vi "Create Wheel Angular Velocity Row.vi"(8 "error in (no error)":errorcluster, 10 "steering angle (rad)":dbl, 11 "mecanum wheel in":refnum<class "NI_Robotics_Mecanum Wheel.lvclass">) -> (0 "error out":errorcluster, 2 "wheel angular velocity row":dbl[](array[numeric]), 3 "mecanum wheel out":refnum<class "NI_Robotics_Mecanum Wheel.lvclass">)   [LabVIEW 2017, in "NI_Robotics_Mecanum Wheel.lvclass"]
uses:
  <vilib>/robotics/Steering/Mecanum Wheel/NI_Robotics_Mecanum Wheel.lvclass
  c:/Program Files (x86)/National Instruments/LabVIEW 2017/vi.lib/robotics/Steering/Wheel/NI_Robotics_Wheel.lvclass
  <vilib>/robotics/Steering/Wheel/NI_Robotics_Wheel.lvclass/NI_Robotics_Wheel.ctl
  <vilib>/robotics/Steering/Mecanum Wheel/NI_Robotics_Mecanum Wheel.lvclass/NI_Robotics_Mecanum Wheel.ctl
  <vilib>/robotics/Steering/Wheel/NI_Robotics_Wheel.lvclass
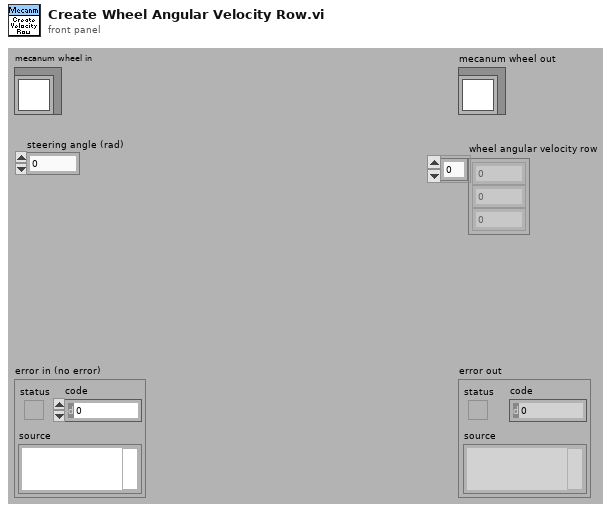
[diagram p1: front panel]
types:
  T1 = typedef "NI_Matrix.lvlib/RealMatrix.ctl" = dbl[][]
  T2 = typedef "NI_Robotics_Mecanum Wheel.lvclass/Roller Orientation.ctl" = u16
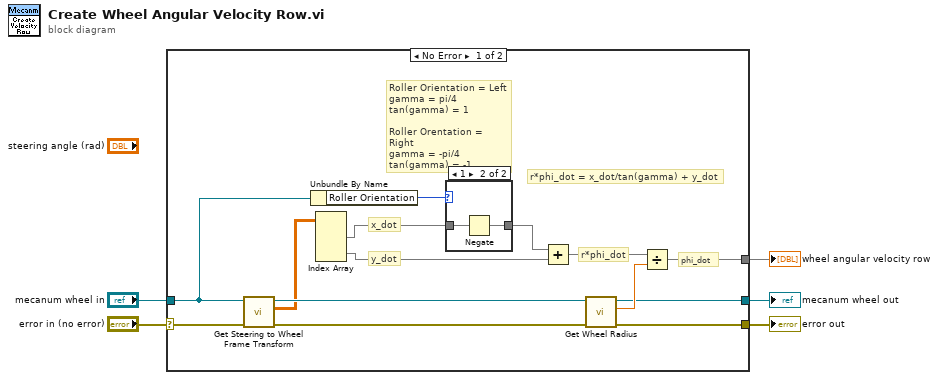
[diagram p0: block diagram]
diagram:
  n1 = case shown="No Error" "error in (no error)" {
    selector: "error in (no error)" -> [w8 w24]
    tunnel: [w15 w24] -> w4
    tunnel: "mecanum wheel in" -> [w10 w23]
    tunnel: [w14 w23] -> w2
    tunnel: [w16 _] -> w1
    frame No Error {
      # "r*phi_dot = x_dot/tan(gamma) + y_dot"
      # "phi_dot"
      # "r*phi_dot"
      # "Roller Orientation = Left\ngamma = pi/4\ntan(gamma) = 1\n\nRoller Orentation = Right\ngamma = -pi/4\ntan(gamma) = -1"
      # "y_dot"
      # "x_dot"
      n2 = call <vilib>:"Get Steering to Wheel Frame Transform.vi"("error in (no error)"=w8, "wheel in"=w10) -> ("error out"=w7:errorcluster, "steering to wheel frame transform"=w6:T1, "wheel out"=w9:refnum<class "NI_Robotics_Mecanum Wheel.lvclass">)  [unwired: 7 in]
      n3 = Unbundle By Name(w10) -> ("Roller Orientation"=w12:T2)
      n4 = Index Array(array=w6) -> (element #1=w13:dbl[], element #2=w19:dbl[])  [unwired: 4 in]
      n5 = case shown="1" w12 {
        tunnel: w13 -> [w20 w22]
        tunnel: [w20 w21] -> w11
        frame 0, Default {
        }
        frame 1 {
          n6 = Negate(x=w22) -> (-x=w21:dbl[])
        }
      }
      n7 = Add(x=w11, y=w19) -> (x+y=w18:dbl[])
      n8 = call <vilib>:"Get Wheel Radius.vi"("error in (no error)"=w7, "wheel in"=w9) -> ("error out"=w15:errorcluster, "wheel radius"=w17:dbl, "wheel out"=w14:refnum<class "NI_Robotics_Mecanum Wheel.lvclass">)  [unwired: 7 in]
      n9 = Divide(x=w18, y=w17) -> (x/y=w16:dbl[])
    }
    frame Error {
    }
  }
  "error out" <- w4
  "mecanum wheel out" <- w2
  "wheel angular velocity row" <- w1
